vi "FilterByColor.vi"(10 "Color":T1, 11 "Products In":refnum<class "Product.lvclass">[](array[class])) -> (3 "Filtered Products":refnum<class "Product.lvclass">[](array[class]))   [LabVIEW 2018, in "ProductFilter.lvclass"]
uses:
  ProductFilter.lvclass
  Product/Product.lvclass
  Product/Color.ctl
  Product/Product.lvclass/Product.ctl
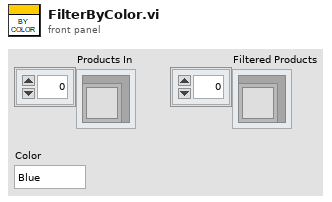
[diagram p1: front panel]
types:
  T1 = typedef "Product.lvclass/Color.ctl" = enum16{"Blue", "Green", "Red"}
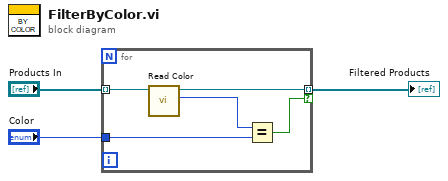
[diagram p0: block diagram]
diagram:
  n1 = for {
    tunnel: "Products In" -> [w8] mode=indexing
    tunnel: [w7] -> w2 mode=indexing if=w4
    tunnel: "Color" -> [w6]
    n2 = call "Read Color.vi"("Product In"=w8) -> ("Color"=w5:T1, "Product Out"=w7:refnum<class "Product.lvclass">)  [unwired: 9 in]
    n3 = Equal?(x=w5, y=w6) -> (x = y?=w4:bool)
  }
  "Filtered Products" <- w2
